vi "SeCrTs-RD NS Receiver.vi"(8 "error in":errorcluster) -> (0 "error out":errorcluster)   [LabVIEW 2022 SP3]
uses:
  Globals/SeCrTs-RD globals.vi
  <resource>/objmgr/ni.dex.rc
panel:
  out "x":u32
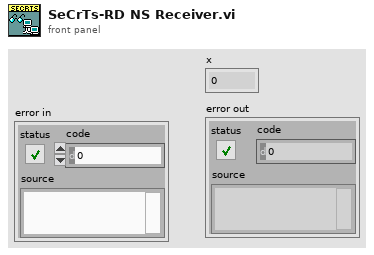
[diagram p1: front panel]
types:
  T1 = cluster{"In Progress":bool, "reader url":refnum<k21>}
  T2 = enum16{"Initialize", "Wait for connection", "Send data", "Exit", "Receive Data"}
  T3 = cluster{"AI_V_Data":waveform(dbl)[][], "AI_C_Data":waveform(dbl)[][], "AO_Data":waveform(dbl)[][], "DO_Data":waveform(dbl)[][], "DI_Data":digitalwaveform[][], "ACC_Data":waveform(dbl)[][], "TC Data":waveform(dbl)[][], "Drive_A_C":waveform(dbl)[][], "Drive_A_D":waveform(dbl)[][], "Drive_L_C":waveform(dbl)[][], "Drive_L_D":waveform(dbl)[][]}
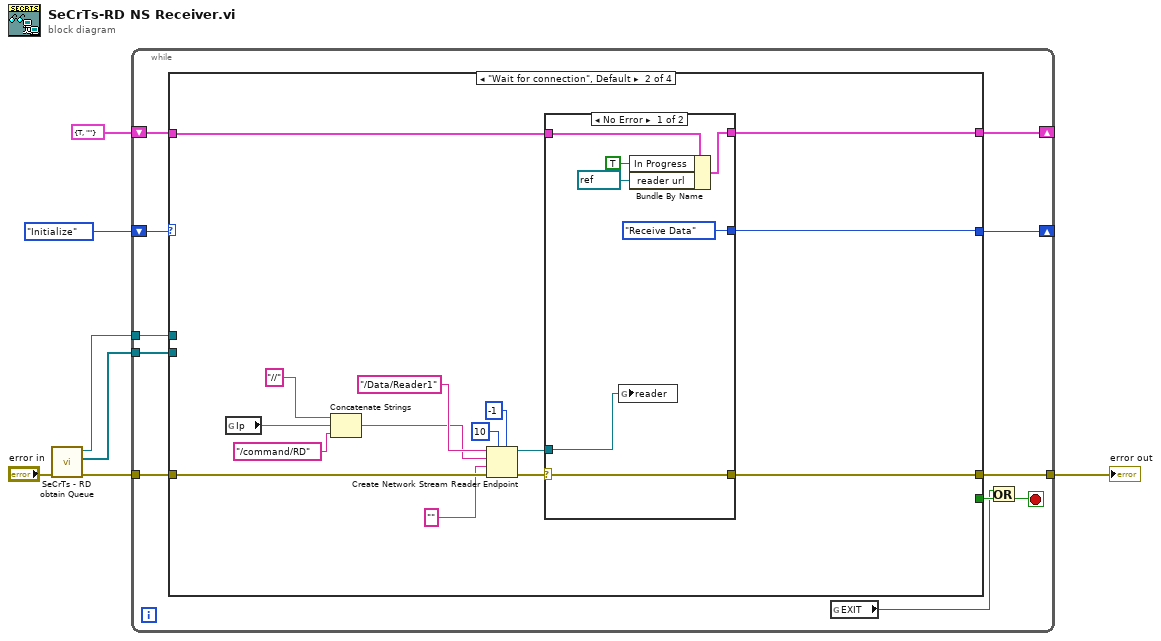
[diagram p0: block diagram]
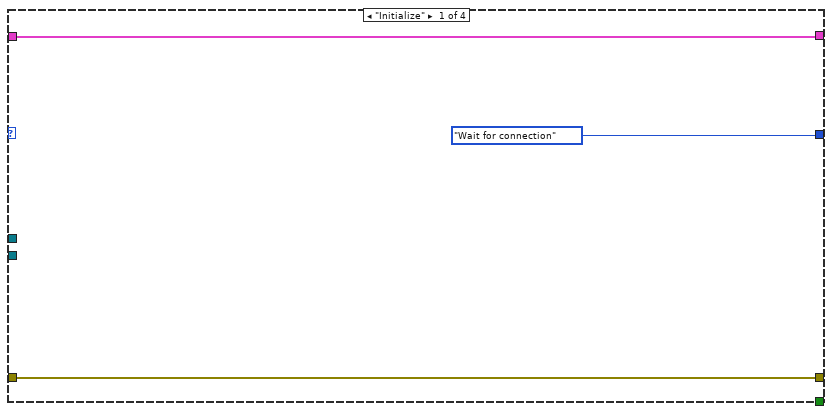
[diagram p2: hidden frame]
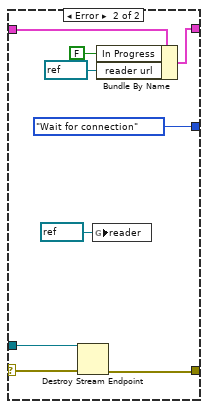
[diagram p3: hidden frame]
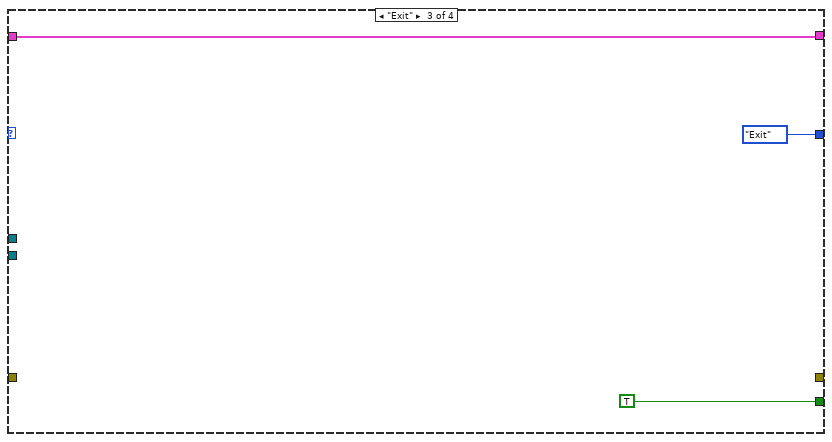
[diagram p4: hidden frame]
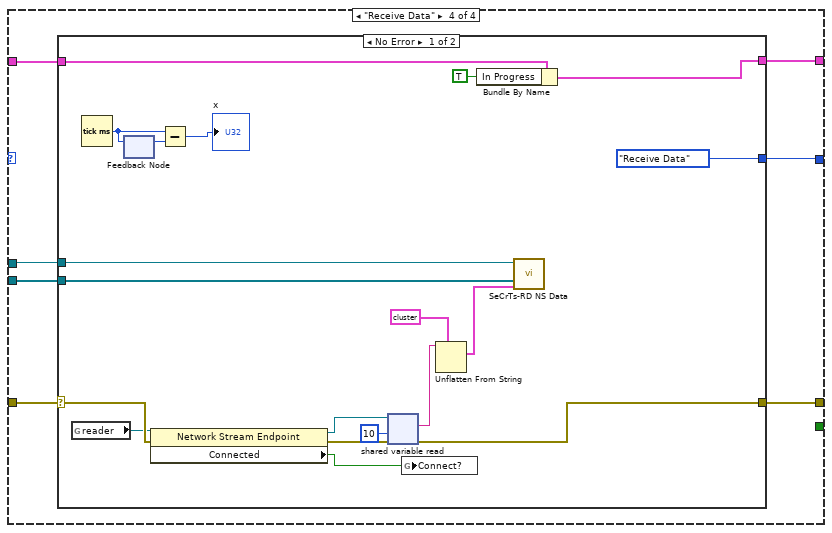
[diagram p5: hidden frame]
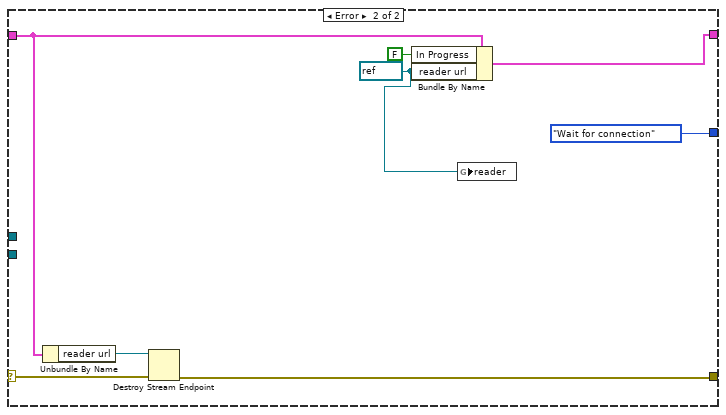
[diagram p6: hidden frame]
diagram:
  n1 = call "SeCrTs - RD obtain Queue.vi"("error in"="error in") -> ("error out"=w4:errorcluster, "Analog Queue"=w2:refnum<queue>[], "DI Data Queue"=w3:refnum<queue>)  [unwired: 8 in]
  n2 = while {
    shift-right: [w16] -> _
    shift-left: T2."Initialize" -> [w18]
    shift-right: [w14] -> _
    shift-left: T1 {"In Progress"=TRUE, "reader url"=""} -> [w15]
    tunnel: w4 -> [w13]
    tunnel: [w12] -> w5
    tunnel: w3 -> [w11]
    tunnel: w2 -> [w8]
    stop <- w10 stop-if-true
    n3 = case shown="\"Wait for connection\", Default" w18 {
      tunnel: [_ _ TRUE _] -> w17
      tunnel: [T2."Wait for connection" w32 T2."Exit" w59] -> w16
      tunnel: w15 -> [w21 w36 w54 w62]
      tunnel: [w21 w35 w54 w60] -> w14
      tunnel: w13 -> [w19 w34 _ w61]
      tunnel: [w19 w33 _ w58] -> w12
      tunnel: w11 -> [_ _ _ w57]
      tunnel: w8 -> [_ _ _ w56]
      frame "Initialize" {
      }
      frame "Wait for connection", Default {
        n4 = global read "SeCrTs-RD globals.vi" "Ip"() -> (w22:string)
        n5 = Concatenate Strings("//" ("string"), w22, "/command/RD" ("reader url")) -> (w24:string)
        n6 = Create Network Stream Reader Endpoint(5:-1 ("timeout in ms (-1)"), 7:10 ("reader buffer size"), 8:w34, 9:"", 10:w24, 11:"/Data/Reader1" ("writer name")) -> (0:w29:errorcluster, 3:w30:refnum<k21>)  [unwired: 1 in]
        n7 = case shown="No Error" w29 {
          selector: w29 -> [w40 w48]
          tunnel: w36 -> [w43 w52]
          tunnel: w30 -> [w38 w49]
          tunnel: [w41 w51] -> w35
          tunnel: [w40 w47] -> w33
          tunnel: [T2."Receive Data" T2."Wait for connection"] -> w32
          frame No Error {
            n8 = global write "SeCrTs-RD globals.vi" "reader"(w38) -> ()
            n9 = Bundle By Name(cluster=w43, "In Progress"=TRUE, "reader url"=refnum<k21> refnum) -> (w41:T1)
          }
          frame Error {
            n10 = Destroy Stream Endpoint(8:w48, 11:w49) -> (0:w47:errorcluster)
            n11 = global write "SeCrTs-RD globals.vi" "reader"(refnum<k21> refnum ("reader")) -> ()
            n12 = Bundle By Name(cluster=w52, "In Progress"=FALSE, "reader url"=refnum<k21> refnum) -> (w51:T1)
          }
        }
      }
      frame "Exit" {
      }
      frame "Receive Data" {
        n13 = case shown="No Error" w61 {
          selector: w61 -> [w76 w84]
          tunnel: w62 -> [w81 w87]
          tunnel: [w80 w89] -> w60
          tunnel: [T2."Receive Data" T2."Wait for connection"] -> w59
          tunnel: [w73 w83] -> w58
          tunnel: w57 -> [w68 _]
          tunnel: w56 -> [w63 _]
          frame No Error {
            n14 = global read "SeCrTs-RD globals.vi" "reader"() -> (w74:refnum<k21>)
            n15 = Tick Count (ms)() -> (millisecond timer value=w70:u32)
            n16 = feedback-in #1(w70) -> ()
            n17 = feedback #1() -> (w71:u32)  [unwired: 1 in]
            n18 = property class="Network Stream Endpoint"(reference=w74, error in=w76) -> (reference out=w78:refnum<k21>, error out=w75:errorcluster, "Connected"=w72:bool)
            n19 = Subtract(x=w70, y=w71) -> (x-y=→"x":u32)
            n20 = shared-variable-read(w78, w75, 10 ("timeout ms (-1)")) -> (w73:errorcluster, w67:string)  [unwired: 2 out]
            n21 = global write "SeCrTs-RD globals.vi" "Connect?"(w72) -> ()
            n22 = Unflatten From String(type=T3 data[101848B] ("data out"), binary string=w67) -> (value=w65:T3)  [unwired: 3 in, 2 out]
            n23 = Bundle By Name(cluster=w81, "In Progress"=TRUE) -> (w80:T1)
            n24 = call "SeCrTs-RD NS Data.vi"("data out"=w65, "Array"=w63, "Queue in"=w68) -> ()  [unwired: 9 in]
          }
          frame Error {
            w82 = refnum<k21> refnum ("reader url")
            n25 = Unbundle By Name(w87) -> ("reader url"=w86:refnum<k21>)
            n26 = Destroy Stream Endpoint(8:w84, 11:w86) -> (0:w83:errorcluster)
            n27 = Bundle By Name(cluster=w87, "In Progress"=FALSE, "reader url"=w82) -> (w89:T1)
            n28 = global write "SeCrTs-RD globals.vi" "reader"(w82) -> ()
          }
        }
      }
    }
    n29 = global read "SeCrTs-RD globals.vi" "EXIT"() -> (w9:bool)
    n30 = Or(x=w9, y=w17) -> (x .or. y?=w10:bool)
  }
  "error out" <- w5
